vi "Set BAUD.vi"(8 "error in (no error)":errorcluster, 10 "Serial Settings:Baud Rate":u32, 11 "Sensor General Class in":refnum<class "Sensor General Class.lvclass">) -> (0 "error out":errorcluster, 3 "Sensor General Class out":refnum<class "Sensor General Class.lvclass">)   [LabVIEW 2020, in "Sensor General Class.lvclass"]
uses:
  Sensor General Class.lvclass
  Sensor General Class.lvclass/Sensor General Class.ctl
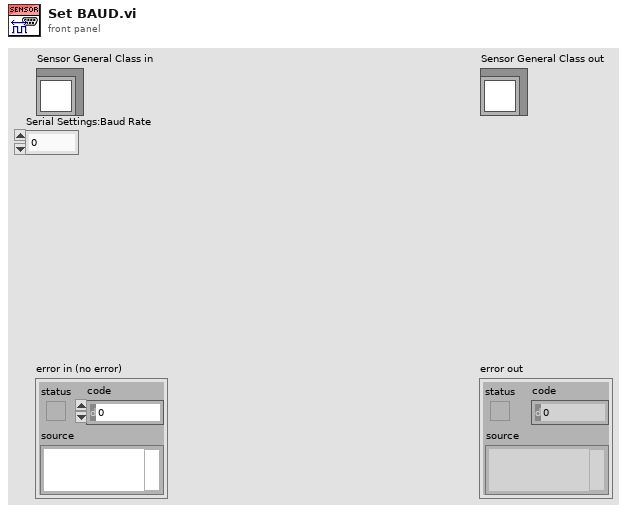
[diagram p1: front panel]
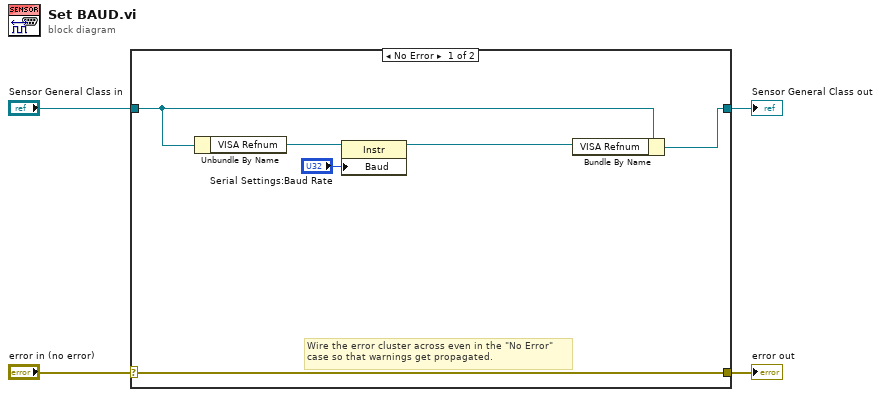
[diagram p0: block diagram]
diagram:
  n1 = case shown="No Error" "error in (no error)" {
    selector: "error in (no error)" -> [w10 w12]
    tunnel: [w10 w12] -> w3
    tunnel: [w8 w11] -> w1
    tunnel: "Sensor General Class in" -> [w9 w11]
    frame No Error {
      # "Wire the error cluster across even in the \"No Error\"\ncase so that warnings get propagated."
      n2 = Unbundle By Name(w9) -> ("VISA Refnum"=w7:refnum<visa-resource-name>)
      n3 = property class="Instr"(reference=w7, "Baud"="Serial Settings:Baud Rate") -> (reference out=w6:refnum<visa-resource-name>)  [unwired: 1 in, 1 out]
      n4 = Bundle By Name(cluster=w9, "VISA Refnum"=w6) -> (w8:refnum<class "Sensor General Class.lvclass">)
    }
    frame Error {
    }
  }
  "error out" <- w3
  "Sensor General Class out" <- w1
